vi "test_definitions_module.vi"() -> ()   [LabVIEW 2015]
panel:
  out "Mode":string
  in  "Mode":T1(ring)
  out "Total test time":dbl format="%.2f"
  out "overlap":dbl format="%.2f"
  in  "Delay":dbl min=0.0 format="%.2f"
  out "19572 test time":dbl format="%.2f"
  out "19052 test time":dbl format="%.2f"
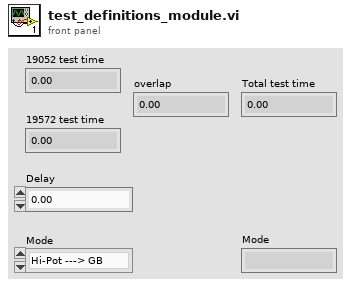
[diagram p1: front panel]
types:
  T1 = enum16{"Hi-Pot ---> GB", "GB ---> Hi-Pot", "Hi-Pot only", "GB only"}
  T2 = cluster{"steps":u16[], "times":string[], "active steps":u16, "modes":string[], "Total time":dbl, "CONT.?":bool}
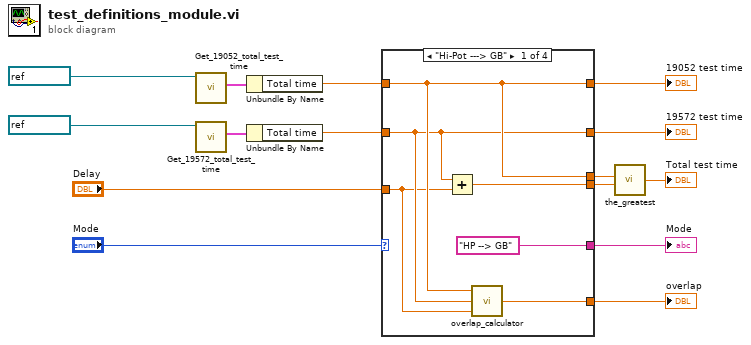
[diagram p0: block diagram]
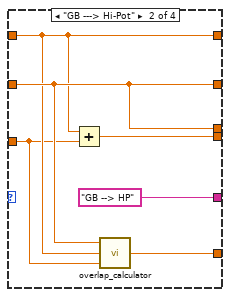
[diagram p2: hidden frame]
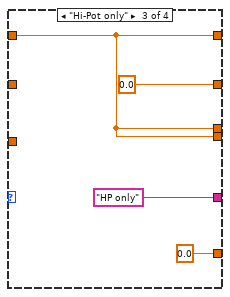
[diagram p3: hidden frame]
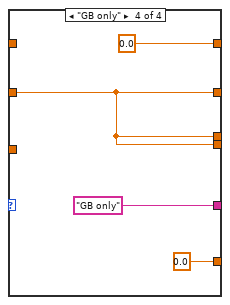
[diagram p4: hidden frame]
diagram:
  n1 = call "Get_19052_total_test_time.vi"("VISA resource in"=refnum<visa-resource-name> "COM5" ("VISA resource in 19052")) -> ("Data"=w12:T2)  [unwired: 8 in, 2 out]
  n2 = call "Get_19572_total_test_time.vi"("VISA resource in"=refnum<visa-resource-name> "COM6" ("VISA resource in 19572")) -> ("Data"=w13:T2)  [unwired: 8 in, 2 out]
  n3 = Unbundle By Name(w12) -> ("Total time"=w4:dbl)
  n4 = Unbundle By Name(w13) -> ("Total time"=w3:dbl)
  n5 = case shown="\"Hi-Pot ---> GB\"" "Mode" {
    tunnel: w4 -> [w18 w23 w29 _]
    tunnel: w3 -> [w17 w24 _ w33]
    tunnel: "Delay" -> [w16 w22 _ _]
    tunnel: [w21 w27 w29 w33] -> w11
    tunnel: [w18 w24 w29 w33] -> w10
    tunnel: [w18 w23 w29 0.0] -> w8
    tunnel: [w17 w24 0.0 w33] -> w7
    tunnel: ["HP --> GB" "GB --> HP" "HP only" "GB only"] -> w6
    tunnel: [w19 w25 0.0 0.0] -> w1
    frame "Hi-Pot ---> GB" {
      n6 = Add(x=w17, y=w16) -> (x+y=w21:dbl)
      n7 = call "overlap_calculator.vi"("T1"=w18, "T2"=w17, "D"=w16) -> ("overlap"=w19:dbl)  [unwired: 4 in]
    }
    frame "GB ---> Hi-Pot" {
      n8 = Add(x=w23, y=w22) -> (x+y=w27:dbl)
      n9 = call "overlap_calculator.vi"("T1"=w24, "T2"=w23, "D"=w22) -> ("overlap"=w25:dbl)  [unwired: 4 in]
    }
    frame "Hi-Pot only" {
    }
    frame "GB only" {
    }
  }
  "19052 test time" <- w8
  "19572 test time" <- w7
  "overlap" <- w1
  "Mode" <- w6
  n10 = call "the_greatest.vi"("A"=w10, "B"=w11) -> ("max"=→"Total test time":dbl)  [unwired: 6 in]
